vi "niRFUtil MT UTIL Resampling Factors.vi"(0 "resampling factor":dbl, 5 "initial sample offset":dbl, 11 "error in (no error)":errorcluster) -> (4 "resampling mode":T1(ring), 6 "fractional factor":dbl format="%#_6p", 8 "integer factor":i32 format="%.0p", 15 "error out":errorcluster)   [LabVIEW 2015, in "niRFUtil.lvlib"]
uses:
  niRFUtil.lvlib
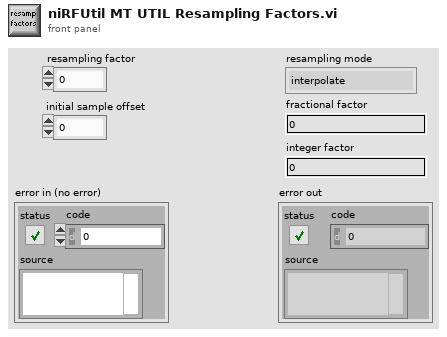
[diagram p1: front panel]
types:
  T1 = enum16{"interpolate", "2-stage interpolate", "decimate", "2-stage decimate", "integer interpolate", "integer decimate", "no resampling"}
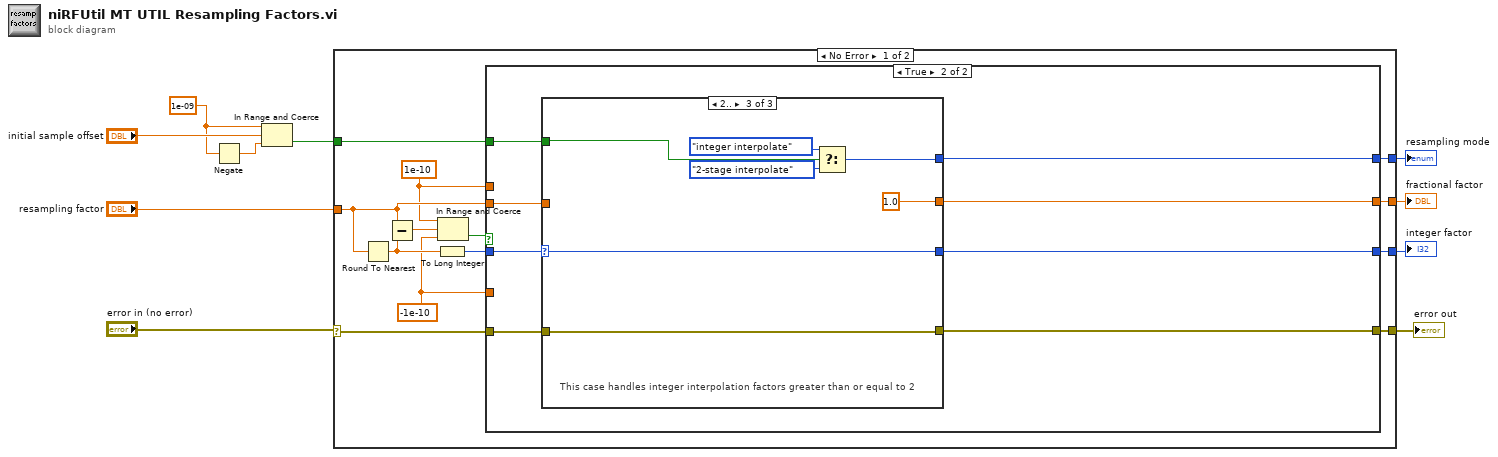
[diagram p0: block diagram]
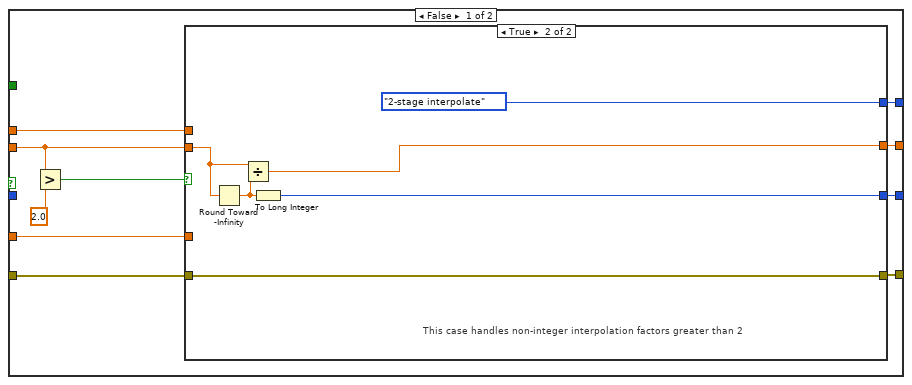
[diagram p2: hidden frame]
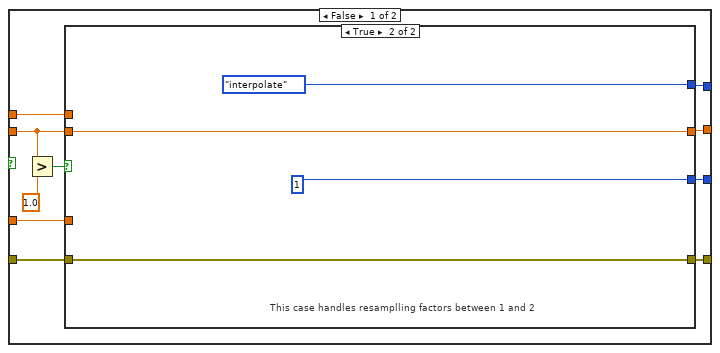
[diagram p3: hidden frame]
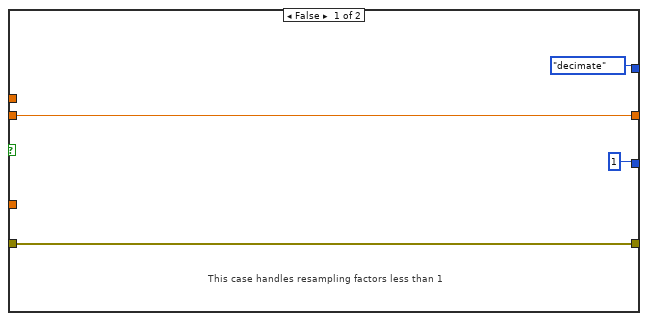
[diagram p4: hidden frame]
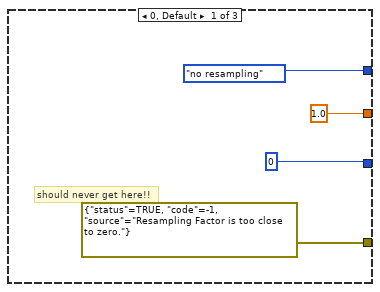
[diagram p5: hidden frame]
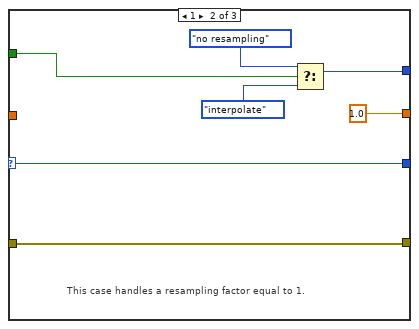
[diagram p6: hidden frame]
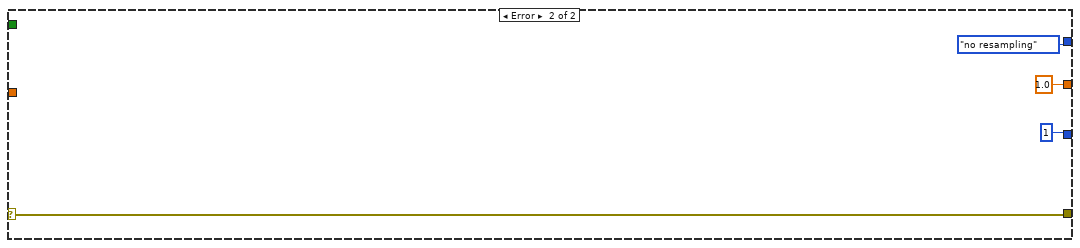
[diagram p7: hidden frame]
diagram:
  w3 = 1e-09 ("upper limit")
  n1 = Negate(x=w3) -> (-x=w2:dbl)
  n2 = In Range and Coerce(upper limit=w3, x="initial sample offset", lower limit=w2) -> (In Range?=w1:bool)  [unwired: 1 out]
  n3 = case shown="No Error" "error in (no error)" {
    selector: "error in (no error)" -> [w16 w87]
    tunnel: [w20 T1."no resampling"] -> w10
    tunnel: [w19 1] -> w9
    tunnel: "resampling factor" -> [w17 _]
    tunnel: [w15 w87] -> w6
    tunnel: [w14 1.0 ("resampling factor")] -> w5
    tunnel: w1 -> [w11 _]
    frame No Error {
      w12 = -1e-10 ("lower limit")
      w13 = 1e-10 ("upper limit")
      n4 = Round To Nearest(number=w17) -> (nearest integer value=w21:dbl)
      n5 = Subtract(x=w17, y=w21) -> (x-y=w23:dbl)
      n6 = To Long Integer(number=w21) -> (32bit integer=w18:i32)
      n7 = In Range and Coerce(upper limit=w13, x=w23, lower limit=w12) -> (In Range?=w22:bool)  [unwired: 1 out]
      n8 = case shown="True" w22 {
        tunnel: w18 -> [_ w64]
        tunnel: [w32 w65] -> w20
        tunnel: [w29 w63] -> w19
        tunnel: w17 -> [w31 w58]
        tunnel: w16 -> [w27 w62]
        tunnel: [w26 w61] -> w15
        tunnel: [w28 w59] -> w14
        tunnel: w13 -> [w25 _]
        tunnel: w12 -> [w24 _]
        tunnel: w11 -> [_ w60]
        frame False {
          n9 = Greater?(x=w31, y=2.0) -> (0:w30:bool)
          n10 = case shown="True" w30 {
            tunnel: [w40 T1."2-stage interpolate"] -> w32
            tunnel: w31 -> [w39 w54]
            tunnel: [w41 w56] -> w29
            tunnel: [w38 w53] -> w28
            tunnel: w27 -> [w37 w52]
            tunnel: [w36 w52] -> w26
            tunnel: w25 -> [w35 _]
            tunnel: w24 -> [w34 _]
            frame False {
              n11 = Greater?(x=w39, y=1.0) -> (0:w42:bool)
              n12 = case shown="True" w42 {
                tunnel: [1 1] -> w41
                tunnel: [T1."decimate" T1."interpolate"] -> w40
                tunnel: w39 -> [w46 w49]
                tunnel: [w46 w49] -> w38
                tunnel: w37 -> [w44 w48]
                tunnel: [w44 w48] -> w36
                tunnel: w35 -> [_ _]
                tunnel: w34 -> [_ _]
                frame False {
                  # "This case handles resampling factors less than 1"
                }
                frame True {
                  # "This case handles resamplling factors between 1 and 2"
                }
              }
            }
            frame True {
              # "This case handles non-integer interpolation factors greater than 2"
              n13 = Round Toward -Infinity(1:w54) -> (0:w55:dbl)
              n14 = Divide(x=w54, y=w55) -> (x/y=w53:dbl)
              n15 = To Long Integer(number=w55) -> (32bit integer=w56:i32)
            }
          }
        }
        frame True {
          n16 = case shown="2.." w64 {
            selector: w64 -> [_ w76 w77]
            tunnel: [T1."no resampling" w72 w81] -> w65
            tunnel: [0 w76 w77] -> w63
            tunnel: w62 -> [_ w75 w83]
            tunnel: [errorcluster {"status"=TRUE, "code"=-1, "source"="Resampling Factor is too close to zero."} ("error IO") w75 w83] -> w61
            tunnel: w60 -> [_ w71 w79]
            tunnel: [1.0 1.0 1.0] -> w59
            tunnel: w58 -> [_ _ _]
            frame 0, Default {
              # "should never get here!!"
            }
            frame 1 {
              # "This case handles a resampling factor equal to 1."
              n17 = Select(t=T1."no resampling", s=w71, f=T1."interpolate") -> (s? t:f=w72:T1)
            }
            frame 2.. {
              # "This case handles integer interpolation factors greater than or equal to 2"
              n18 = Select(t=T1."integer interpolate", s=w79, f=T1."2-stage interpolate") -> (s? t:f=w81:T1)
            }
          }
        }
      }
    }
    frame Error {
    }
  }
  "resampling mode" <- w10
  "integer factor" <- w9
  "error out" <- w6
  "fractional factor" <- w5
